vi "check Path String and Path Array Reflect.vi"(8 "error in (no error)":errorcluster, 9 "Array":string[](array[string]), 10 "String":string, 11 "Variant Data Manipulation Tests in":refnum<class "Variant Data Manipulation Tests.lvclass">) -> (0 "error out":errorcluster, 3 "Variant Data Manipulation Tests out":refnum<class "Variant Data Manipulation Tests.lvclass">)   [LabVIEW 2017, in "Variant Data Manipulation Tests.lvclass"]
uses:
  Variant Data Manipulation Tests.lvclass
  Source/Variant Data Manipulation.lvlib
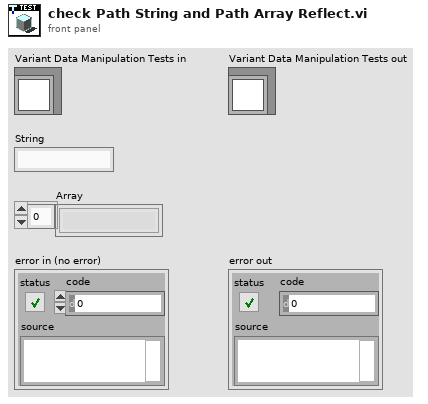
[diagram p1: front panel]
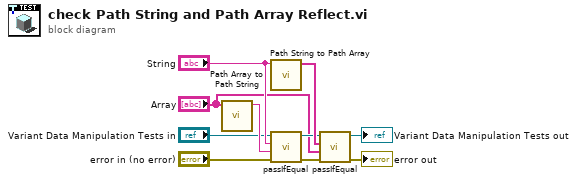
[diagram p0: block diagram]
diagram:
  n1 = call "Path Array to Path String.vi"("path array"="Array") -> ("path"=w10:string)  [unwired: 10 in]
  n2 = call "Path String to Path Array.vi"("Path String"="String") -> ("Path Array"=w9:string[])  [unwired: 9 in, 1 out]
  n3 = call-dynamic "passIfEqual.vi"("error in (no error)"="error in (no error)", "y"=w10, "x"="String", "TestCase in"="Variant Data Manipulation Tests in") -> ("error out"=w3:errorcluster, "TestCase out"=w6:refnum<class "Variant Data Manipulation Tests.lvclass">)  [unwired: 6 in]
  n4 = call-dynamic "passIfEqual.vi"("error in (no error)"=w3, "y"="Array", "x"=w9, "TestCase in"=w6) -> ("error out"=→"error out":errorcluster, "TestCase out"=→"Variant Data Manipulation Tests out":refnum<class "Variant Data Manipulation Tests.lvclass">)  [unwired: 6 in]
